vi "Send New Command Processor Status.vi"(7 "Message Priority (Normal)":T6=enum."Normal", 8 "error in (no error)":errorcluster, 10 "Command Processor Status":T1, 11 "Message Enqueuer":refnum<class "Message Enqueuer.lvclass">) -> (0 "error out":errorcluster, 3 "Message Enqueuer out":refnum<class "Message Enqueuer.lvclass">)   [LabVIEW 2013, in "System.lvlib" / "New Command Processor Status Msg.lvclass"]
doc: "This VI sends the message to an actor."
uses:
  New Command Processor Status Msg.lvclass
  <vilib>/ActorFramework/Message Enqueuer/Message Enqueuer.lvclass
  <vilib>/ActorFramework/Message Enqueuer/Message Priority.ctl
  Command Processor/Command Processor Status.ctl
  Current Previous State Status.ctl
  State Status.ctl
  Command Processor/Command/Command Status.ctl
  Command Processor/Command/State Status.ctl
  New Command Processor Status Msg.lvclass/New Command Processor Status Msg.ctl
  <vilib>/ActorFramework/Message Enqueuer/Message Enqueuer.lvclass/Message Enqueuer.ctl
  <vilib>/ActorFramework/Message Priority Queue/Priority Enqueue.vi
  Command Processor/Command/Command.lvclass
  Command Processor/Command Processor.lvclass
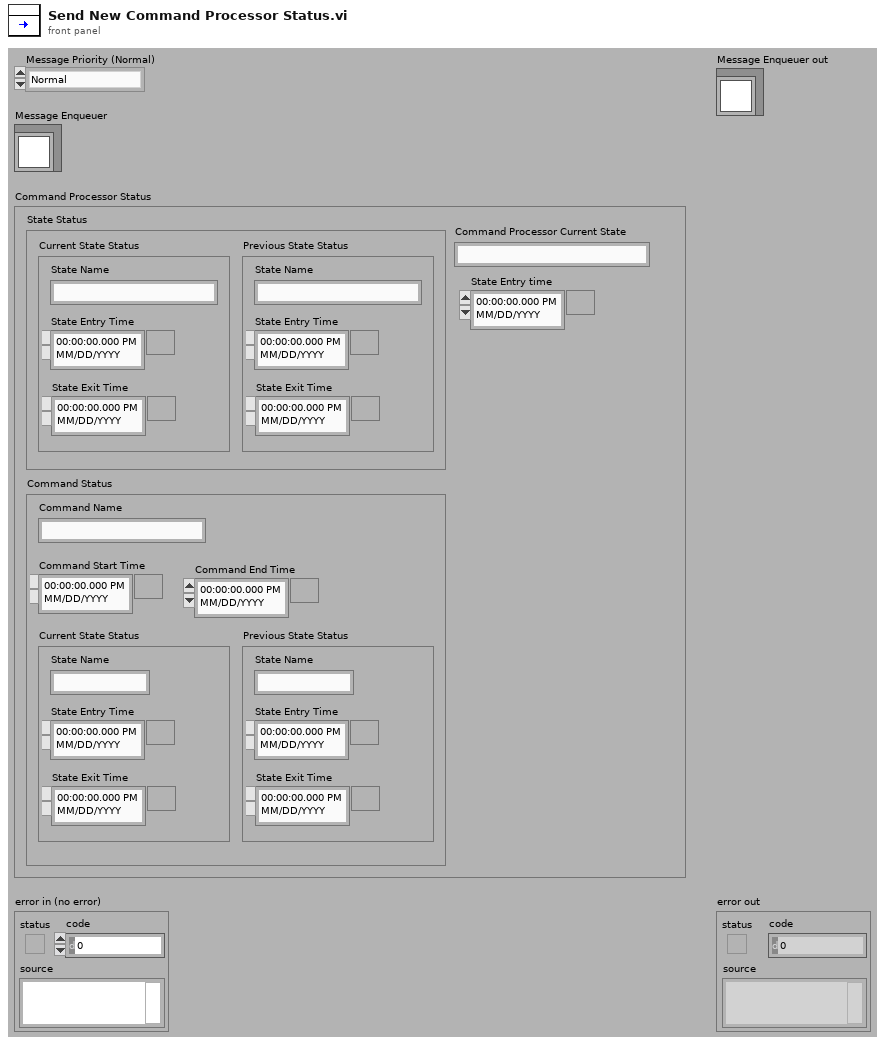
[diagram p1: front panel]
types:
  T1 = typedef "Command Processor.lvlib/Command Processor.lvclass/Command Processor Status.ctl" = cluster{"State Entry time":timestamp, "State Status":T2, "Command Processor Current State":string, "Command Status":T4}
  T2 = typedef "Current Previous State Status.ctl" = cluster{"Current State Status":T3, "Previous State Status":T3}
  T3 = typedef "State Status.ctl" = cluster{"State Name":string, "State Entry Time":timestamp, "State Exit Time":timestamp}
  T4 = typedef "Command Processor.lvlib/Command.lvlib/Command.lvclass/Command Status.ctl" = cluster{"Command Name":string, "Current State Status":T5, "Command Start Time":timestamp, "Command End Time":timestamp, "Previous State Status":T5}
  T5 = typedef "Command Processor.lvlib/Command.lvlib/Command.lvclass/State Status.ctl" = cluster{"State Name":string, "State Entry Time":timestamp, "State Exit Time":timestamp}
  T6 = typedef "Actor Framework.lvlib/Message Enqueuer.lvclass/Message Priority.ctl" = enum16{"Low", "Normal", "High"}
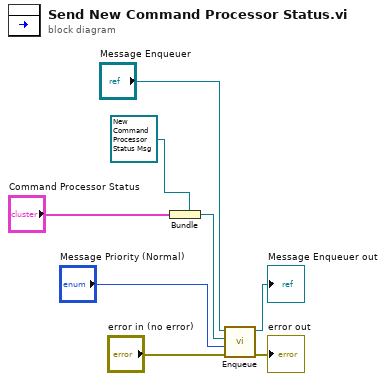
[diagram p0: block diagram]
diagram:
  n1 = Bundle(cluster=refnum<class "New Command Processor Status Msg.lvclass"> refnum ("Object"), "Command Processor Status") -> (w4:refnum<class "New Command Processor Status Msg.lvclass">)
  n2 = call <vilib>:"Enqueue.vi"("error in (no error)"="error in (no error)", "Message Priority (Normal)"="Message Priority (Normal)", "Message"=w4, "Message Enqueuer in"="Message Enqueuer") -> ("error out"=→"error out":errorcluster, "Message Enqueuer out"=→"Message Enqueuer out":refnum<class "Message Enqueuer.lvclass">)  [unwired: 6 in]
